vi "SPC_X-bar and Chart Sample.vi"() -> ()   [LabVIEW 2014]
uses:
  <vilib>/addons/SPC/NI_DSC_SPC.lvlib
panel:
  in  "stop":bool
  out "Range Limits":cluster{"UCL":dbl, "CL":dbl, "LCL":dbl} {"UCL" format="%.3f"; "CL" format="%.3f"; "LCL" format="%.3f"}
  out "X-bar Limits":cluster{"UCL":dbl, "CL":dbl, "LCL":dbl} {"UCL" format="%.3f"; "CL" format="%.3f"; "LCL" format="%.3f"}
  out "Range Chart":T1(graph)
  out "X-bar Chart":T1(graph)
  in  "samples X":dbl[][](array[numeric]) format="%.3f"
  # "Sample 1 Row 1\nSample 2 Row 2"
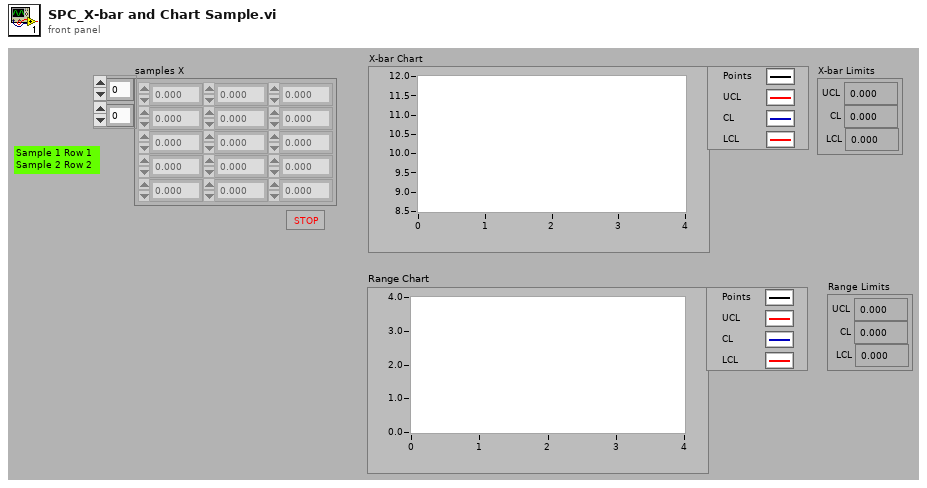
[diagram p1: front panel]
types:
  T1 = cluster{cluster{"starting sample number (0)":i32, "LCL":dbl}[]}[]
  T2 = cluster{"UCLr":dbl, "CLr":dbl, "LCLr":dbl, "standard error":dbl}
  T3 = cluster{"UCLx":dbl, "CLx":dbl, "LCLx":dbl, "standard error":dbl}
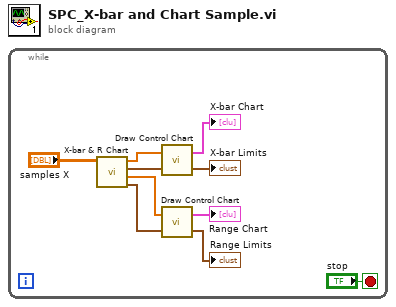
[diagram p0: block diagram]
diagram:
  n1 = while {
    stop <- "stop" stop-if-true
    n2 = call <vilib>:"X-bar & R Chart.vi"("samples X"="samples X") -> ("R chart limits"=w6:T2, "Range R"=w7:dbl[], "X-bar chart limits"=w9:T3, "X-bar"=w8:dbl[])  [unwired: 4 in, 3 out]
    n3 = call <vilib>:"Draw Control Chart.vi"("chart limits"=w9, "points"=w8) -> ("control chart lines"=→"X-bar Limits":cluster{"UCL":dbl, "CL":dbl, "LCL":dbl}, "control chart"=→"X-bar Chart":T1)  [unwired: 2 in]
    n4 = call <vilib>:"Draw Control Chart.vi"("chart limits"=w6, "points"=w7) -> ("control chart lines"=→"Range Limits":cluster{"UCL":dbl, "CL":dbl, "LCL":dbl}, "control chart"=→"Range Chart":T1)  [unwired: 2 in]
  }
